vi "BuildTestFromProjectItem_LibraryWithNestedLibrary_BuildsTestSuiteWithNestedTestSuite.vi"() -> ()   [LabVIEW 2019, in "LVUnitTestBuilderTest.lvlib"]
uses:
  LVUnitTestBuilderTest.lvlib
  LVUnitTestBuilder/LVUnitTestBuilder.lvclass
  TestSuite/TestSuite.lvclass
  TestSuite/TestSuite.lvclass/TestSuite.ctl
  TestSuite/ReadTests.vi
  Test/Test.lvclass
  Assertion/Assertion.lvlib
panel:
  out "error out":errorcluster
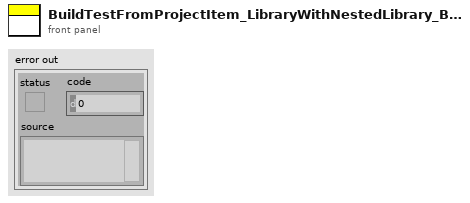
[diagram p1: front panel]
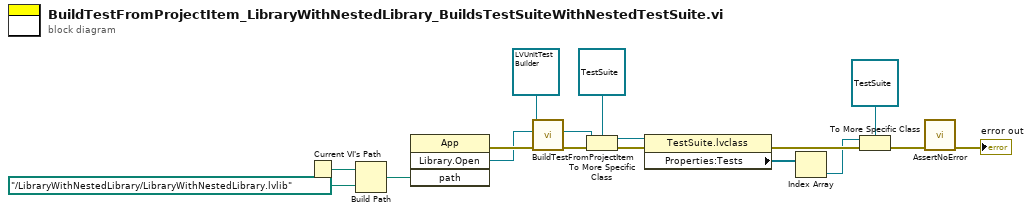
[diagram p0: block diagram]
diagram:
  n1 = Current VI's Path() -> (path=w10:path)
  n2 = Build Path(base path=w10, name or relative path=path "../LibraryWithNestedLibrary/LibraryWithNestedLibrary.lvlib") -> (appended path=w9:path)
  n3 = invoke class="App" method="Library.Open"("path"=w9) -> (error out=w13:errorcluster, "Open Library"=w12:refnum<vi>)  [unwired: 3 in, 2 out]
  n4 = call-dynamic "BuildTestFromProjectItem.vi"("error in (no error)"=w13, "ProjectItem Refnum"=w12, "LVUnitTestBuilder in"=refnum<class "LVUnitTestBuilder.lvclass"> refnum ("LVUnitTestBuilder")) -> ("error out"=w14:errorcluster, "Test"=w16:refnum<class "Test.lvclass">)  [unwired: 6 in, 1 out]
  n5 = To More Specific Class(target class=refnum<class "TestSuite.lvclass"> refnum ("TestSuite.lvclass"), reference=w16, error in=w14) -> (specific class reference=w7:refnum<class "TestSuite.lvclass">, error out=w8:errorcluster)
  n6 = property class="TestSuite.lvclass"(reference=w7, error in=w8) -> (error out=w5:errorcluster, "Properties:Tests"=w6:refnum<class "Test.lvclass">[])  [unwired: 1 out]
  n7 = Index Array(array=w6) -> (element=w4:refnum<class "Test.lvclass">)  [unwired: 1 in]
  n8 = To More Specific Class(target class=refnum<class "TestSuite.lvclass"> refnum ("TestSuite.lvclass"), reference=w4, error in=w5) -> (error out=w1:errorcluster)  [unwired: 1 out]
  n9 = call "AssertNoError.vi"("error in (no error)"=w1) -> ("error out"=→"error out":errorcluster)  [unwired: 10 in]
